vi "Move piece.vi"(8 "error in (no error)":errorcluster, 9 "Destination":T1={"File"=enum."a", "Rank"=enum."4"}, 10 "Source":T1={"File"=enum."a", "Rank"=enum."4"}, 11 "Board in":refnum<class "Board.lvclass">) -> (0 "error out":errorcluster, 1 "Removed piece":refnum<class "Piece.lvclass">, 2 "Destination occupied?":bool, 3 "Board out":refnum<class "Board.lvclass">)   [LabVIEW 2016, in "Chesslib.lvlib" / "Board.lvclass"]
uses:
  Board.lvclass
  typedef/Square.ctl
  typedef/File.ctl
  typedef/Rank.ctl
  Pieces/Piece/Piece.lvclass
  Chesslib.lvlib
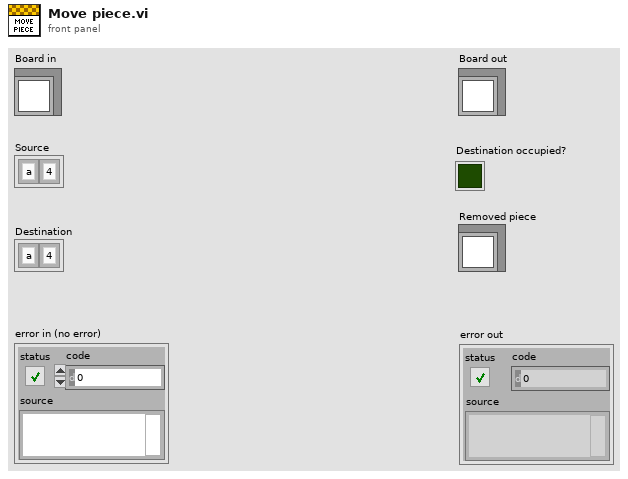
[diagram p1: front panel]
types:
  T1 = typedef "Chesslib.lvlib/Square.ctl" = cluster{"File":T2, "Rank":T3}
  T2 = typedef "Chesslib.lvlib/File.ctl" = enum8{"a", "b", "c", "d", "e", "f", "g", "h"}
  T3 = typedef "Chesslib.lvlib/Rank.ctl" = enum8{"1", "2", "3", "4", "5", "6", "7", "8"}
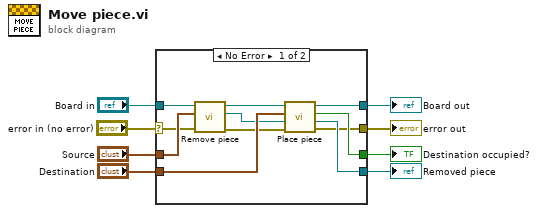
[diagram p0: block diagram]
diagram:
  n1 = case shown="No Error" "error in (no error)" {
    selector: "error in (no error)" -> [w12 w21]
    tunnel: "Board in" -> [w19 w20]
    tunnel: [w18 w20] -> w7
    tunnel: "Source" -> [w17 _]
    tunnel: "Destination" -> [w16 _]
    tunnel: [w15 _] -> w4
    tunnel: [w14 _] -> w3
    tunnel: [w10 w21] -> w1
    frame No Error {
      n2 = call "Remove piece.vi"("error in (no error)"=w12, "Square"=w17, "Board in"=w19) -> ("error out"=w11:errorcluster, "Removed piece"=w9:refnum<class "Piece.lvclass">, "Board out"=w13:refnum<class "Board.lvclass">)  [unwired: 6 in]
      n3 = call "Place piece.vi"("error in (no error)"=w11, "Piece"=w9, "Square"=w16, "Board in"=w13) -> ("error out"=w10:errorcluster, "Removed piece"=w14:refnum<class "Piece.lvclass">, "Square occupied?"=w15:bool, "Board out"=w18:refnum<class "Board.lvclass">)  [unwired: 4 in]
    }
    frame Error {
    }
  }
  "Board out" <- w7
  "Removed piece" <- w3
  "Destination occupied?" <- w4
  "error out" <- w1
